vi "Blackstart Init.vi"(8 "error in":errorcluster, 11 "SCADA in":refnum<class "EMS.lvclass">) -> (0 "error out":errorcluster, 3 "SCADA out":refnum<class "EMS.lvclass">)   [LabVIEW 2018, in "EMS Core.lvlib" / "EMS.lvclass"]
uses:
  EMS.lvclass
  C:/Program Files (x86)/National Instruments/LabVIEW 2018/vi.lib/ActorFramework/Actor/Actor.lvclass
  Controls/Microgrid State.ctl
  EMS.lvclass/EMS.ctl
  <vilib>/ActorFramework/Actor/Actor.lvclass/Actor.ctl
  <vilib>/ActorFramework/Message Enqueuer/Message Enqueuer.lvclass/Message Enqueuer.ctl
  EMS Messages/Return Microgrid State Msg/Return Microgrid State Msg.lvclass/Return Microgrid State Msg.ctl
  <vilib>/ActorFramework/Message Enqueuer/Enqueue.vi
  <vilib>/ActorFramework/Stop Msg/Stop Msg.lvclass
  C:/Program Files (x86)/National Instruments/LabVIEW 2018/vi.lib/ActorFramework/Message/Message.lvclass
  EMS Messages/Return Microgrid State Msg/Return Microgrid State Msg.lvclass
  <vilib>/ActorFramework/Message Priority Queue/Priority Enqueue.vi
  <vilib>/ActorFramework/Actor/Actor.lvclass
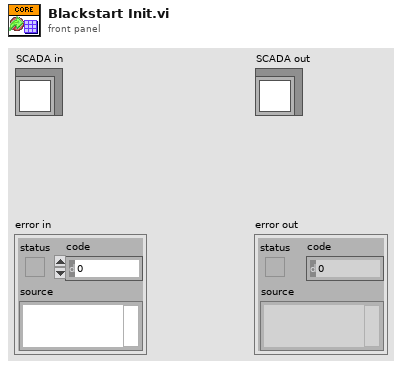
[diagram p1: front panel]
types:
  T1 = typedef "EMS Core.lvlib/EMS.lvclass/Microgrid State.ctl" = enum16{"Discovery", "Commissioning", "Activation", "Blackstart", "OnGrid", "OffGrid", "Island", "Resynchronization", "Manual", "Shutdown", "Stop"}
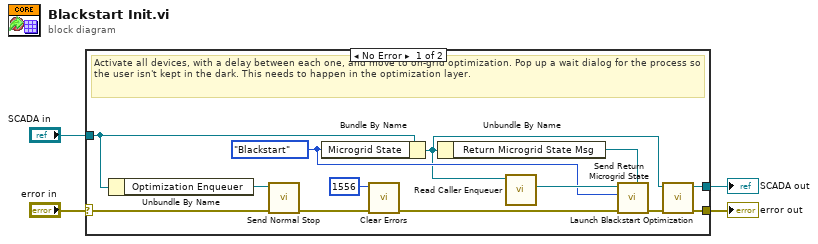
[diagram p0: block diagram]
diagram:
  n1 = case shown="No Error" "error in" {
    selector: "error in" -> [w12 w19]
    tunnel: [w7 w19] -> w3
    tunnel: [w9 w18] -> w1
    tunnel: "SCADA in" -> [w14 w18]
    frame No Error {
      w15 = Microgrid_State."Blackstart" ("Microgrid State")
      # "Activate all devices, with a delay between each one, and move to on-grid optimization. Pop up a wait dialog for the process so the user isn't kept in the dark. This needs to happen in the optimization layer."
      n2 = Unbundle By Name(w14) -> ("Optimization Enqueuer"=w13:refnum<class "Message Enqueuer.lvclass">)
      n3 = call <vilib>:"Send Normal Stop.vi"("error in (no error)"=w12, "Message Enqueuer"=w13) -> ("error out"=w11:errorcluster)  [unwired: 9 in]
      n4 = Bundle By Name(cluster=w14, "Microgrid State"=w15) -> (w10:refnum<class "EMS.lvclass">)
      n5 = call <vilib>:"Clear Errors.vi"("error in (no error)"=w11, "specific error code to clear (0: all)"=1556) -> ("error out"=w6:errorcluster)  [unwired: 4 in, 1 out]
      n6 = Unbundle By Name(w10) -> ("Return Microgrid State Msg"=w16:refnum<class "Return Microgrid State Msg.lvclass">)
      n7 = call <vilib>:"Read Caller Enqueuer.vi"("Actor"=w10) -> ("Caller Enqueuer"=w17:refnum<class "Message Enqueuer.lvclass">)  [unwired: 10 in]
      n8 = call "Send Return Microgrid State.vi"("Message Type"=w16, "error in (no error)"=w6, "Microgrid State"=w15, "Message Enqueuer"=w17) -> ("error out"=w8:errorcluster)  [unwired: 6 in, 1 out]
      n9 = call "Launch Blackstart Optimization.vi"("error in"=w8, "SCADA in"=w10) -> ("error out"=w7:errorcluster, "SCADA out"=w9:refnum<class "EMS.lvclass">)  [unwired: 8 in]
    }
    frame Error {
    }
  }
  "error out" <- w3
  "SCADA out" <- w1
